vi "紀錄.vi"() -> ()   [LabVIEW 2014]
panel:
  in  "stop 2":bool
  in  "stop":bool
  out "number (0 to 1)":dbl
  out "appended array":dbl[][](array[numeric])
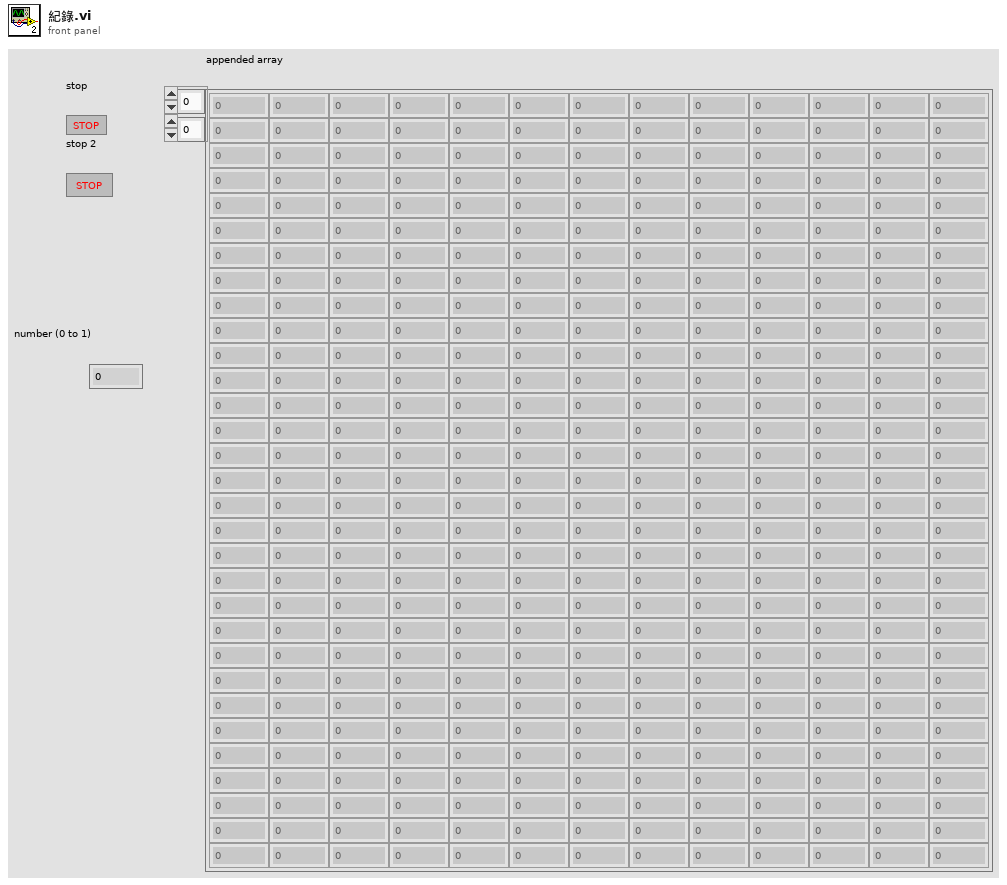
[diagram p1: front panel]
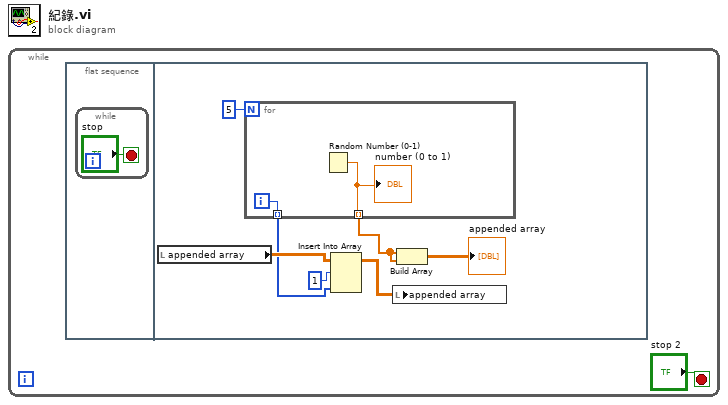
[diagram p0: block diagram]
diagram:
  n1 = while {
    stop <- "stop 2" stop-if-true
    n2 = flat-sequence {
      frame #0 {
        n3 = while {
          stop <- "stop" stop-if-true
        }
      }
      frame #1 {
        n4 = local read "appended array"() -> (w7:dbl[][])
        n5 = for {
          N: 5 -> [_]
          tunnel: [w11] -> w5 mode=indexing
          tunnel: [w10] -> w4 mode=indexing
          i -> [w10]
          n6 = Random Number (0-1)() -> (number: 0 to 1=w11:dbl)
          "number (0 to 1)" <- w11
        }
        n7 = Insert Into Array(array=w7, index (row)=1 ("disabled index (col)"), new element=w4) -> (w6:dbl[][])  [unwired: 1 in]
        n8 = local write "appended array"(w6) -> ()
        n9 = Build Array(w5, w5) -> (→"appended array":dbl[][])
      }
    }
  }
